vi "test_verify_threshold.vi"() -> ()   [LabVIEW 2015]
uses:
  _SubVIs/Advanced/threshold-double.vi
  binary_search.lvlib
panel:
  out "Error?":bool
  in  "Passes":i32=10000
  in  "Elements to Generate":i32=100000
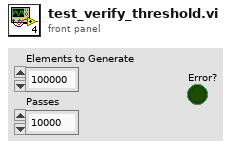
[diagram p1: front panel]
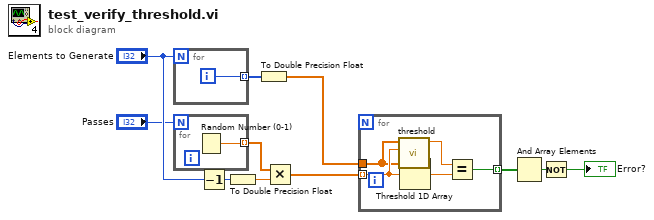
[diagram p0: block diagram]
diagram:
  n1 = for {
    N: "Elements to Generate" -> [_]
    tunnel: [w12] -> w6 mode=indexing
    i -> [w12]
  }
  n2 = for {
    N: "Passes" -> [_]
    tunnel: [w13] -> w5 mode=indexing
    n3 = Random Number (0-1)() -> (number: 0 to 1=w13:dbl)
  }
  n4 = Decrement(x="Elements to Generate") -> (x-1=w3:i32)
  n5 = To Double Precision Float(number=w3) -> (double precision float=w4:dbl)
  n6 = To Double Precision Float(number=w6) -> (double precision float=w7:dbl[])
  n7 = Multiply(x=w5, y=w4) -> (x*y=w8:dbl[])
  n8 = for {
    tunnel: w7 -> [w14]
    tunnel: w8 -> [w18] mode=indexing
    tunnel: [w15] -> w2 mode=indexing
    n9 = call-poly "threshold.vi"("Search"=w18, "Data (dbl) []"=w14) -> ("Index"=w17:dbl)  [unwired: 9 in]
    n10 = Threshold 1D Array(2:w18, 3:w14) -> (0:w16:dbl)  [unwired: 1 in]
    n11 = Equal?(x=w17, y=w16) -> (x = y?=w15:bool)
  }
  n12 = And Array Elements(Boolean array=w2) -> (logical AND=w11:bool)
  n13 = Not(x=w11) -> (.not. x?=→"Error?":bool)
